vi "hw5 counter#1.vi"() -> ()   [LabVIEW 2020]
panel:
  out "1":bool
  out "2":bool
  out "4":bool
  out "8":bool
  out "16":bool
  out "count (binary)":i32 format="%b"
  out "count (hex)":i32 format="%x"
  in  "Count Down":bool
  in  "milliseconds to wait":u32
  in  "Count Up":bool
  out "count (base 10)":i32
  in  "stop":bool
  # "On=1. Off=0\nBinary:"
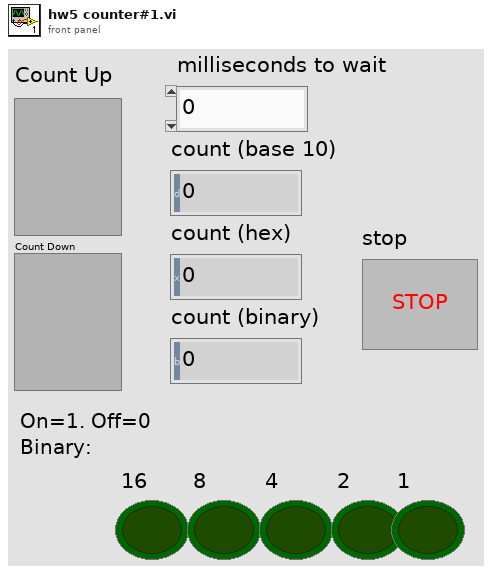
[diagram p1: front panel]
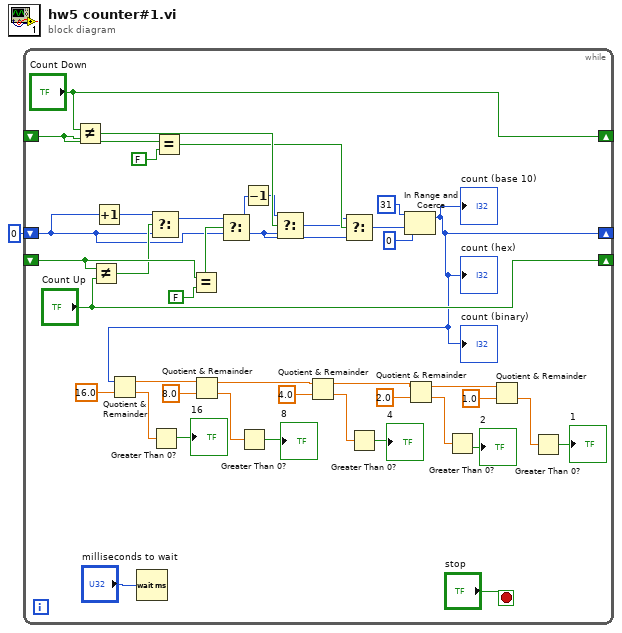
[diagram p0: block diagram]
diagram:
  n1 = while {
    shift-right: [w15] -> _
    shift-left: 0 -> [w23]
    shift-right: ["Count Up"] -> _
    shift-left: _ -> [w35]
    shift-right: ["Count Down"] -> _
    shift-left: _ -> [w29]
    stop <- "stop" stop-if-true
    n2 = Not Equal?(x="Count Down", y=w29) -> (x != y?=w28:bool)
    n3 = Not Equal?(x=w35, y="Count Up") -> (x != y?=w34:bool)
    n4 = Increment(x=w23) -> (x+1=w41:i32)
    n5 = Wait (ms)(milliseconds to wait="milliseconds to wait") -> ()  [unwired: 1 out]
    n6 = Select(t=w41, s=w34, f=w23) -> (s? t:f=w32:i32)
    n7 = Equal?(x=w29, y=FALSE) -> (x = y?=w26:bool)
    n8 = Equal?(x=w35, y=FALSE) -> (x = y?=w33:bool)
    n9 = Select(t=w32, s=w33, f=w23) -> (s? t:f=w22:i32)
    n10 = Decrement(x=w22) -> (x-1=w27:i32)
    n11 = Select(t=w27, s=w28, f=w22) -> (s? t:f=w25:i32)
    n12 = Select(t=w25, s=w26, f=w22) -> (s? t:f=w24:i32)
    n13 = In Range and Coerce(upper limit=31, x=w24, lower limit=0) -> (coerced(x)=w15:i32)  [unwired: 1 out]
    "count (base 10)" <- w15
    "count (hex)" <- w15
    "count (binary)" <- w15
    n14 = Quotient & Remainder(x=w15, y=16.0) -> (x-y*floor(x/y)=w18:dbl, floor(x/y)=w21:dbl)
    n15 = Greater Than 0?(x=w21) -> (x > 0?=→"16":bool)
    n16 = Quotient & Remainder(x=w18, y=8.0) -> (x-y*floor(x/y)=w11:dbl, floor(x/y)=w20:dbl)
    n17 = Greater Than 0?(x=w20) -> (x > 0?=→"8":bool)
    n18 = Quotient & Remainder(x=w11, y=4.0) -> (x-y*floor(x/y)=w7:dbl, floor(x/y)=w13:dbl)
    n19 = Greater Than 0?(x=w13) -> (x > 0?=→"4":bool)
    n20 = Quotient & Remainder(x=w7, y=2.0) -> (x-y*floor(x/y)=w3:dbl, floor(x/y)=w9:dbl)
    n21 = Greater Than 0?(x=w9) -> (x > 0?=→"2":bool)
    n22 = Quotient & Remainder(x=w3, y=1.0) -> (floor(x/y)=w5:dbl)  [unwired: 1 out]
    n23 = Greater Than 0?(x=w5) -> (x > 0?=→"1":bool)
  }
